vi "Tets.vi"() -> ()   [LabVIEW 2025]
panel:
  in  "Color Box 3":u32(colorbox)
  in  "Color Box 2":u32(colorbox)
  in  "Color Box":u32(colorbox)
  in  "stop":bool
  in  "VISA resource name":refnum<visa-resource-name>
  in  "error in (no error)":errorcluster
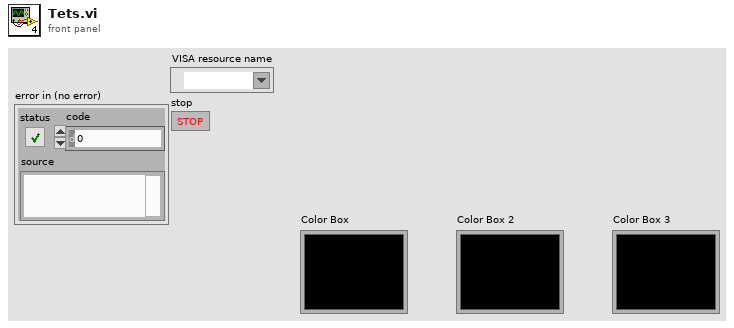
[diagram p1: front panel]
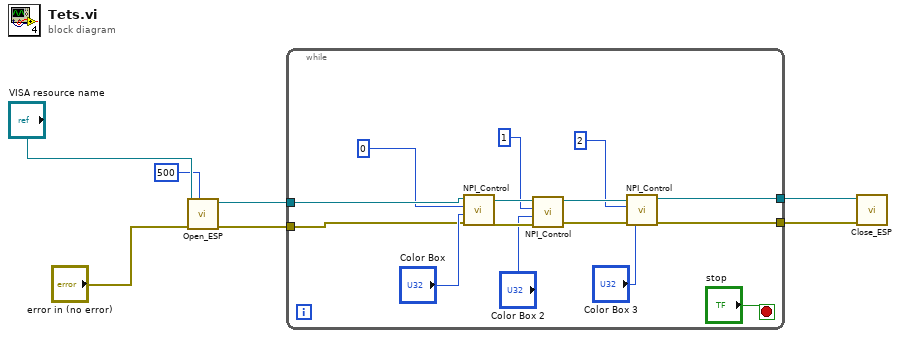
[diagram p0: block diagram]
diagram:
  n1 = call "Open_ESP.vi"("timeout (10sec)"=u32 500, "error in (no error)"="error in (no error)", "VISA resource name"="VISA resource name") -> ("error out"=w3:errorcluster, "VISA resource name out"=w4:refnum<visa-resource-name>)  [unwired: 7 in]
  n2 = while {
    tunnel: w4 -> [w19]
    tunnel: w3 -> [w20]
    tunnel: [w13] -> w2
    tunnel: [w12] -> w1
    stop <- "stop" stop-if-true
    n3 = call "NPI_Control.vi"("error in (no error)"=w20, "Color Box"="Color Box", "No. NeoPixel"=u8 0, "VISA resource name"=w19) -> ("error out"=w16:errorcluster, "VISA resource name out"=w17:refnum<visa-resource-name>)  [unwired: 6 in]
    n4 = call "NPI_Control.vi"("error in (no error)"=w16, "Color Box"="Color Box 2", "No. NeoPixel"=u8 1, "VISA resource name"=w17) -> ("error out"=w11:errorcluster, "VISA resource name out"=w10:refnum<visa-resource-name>)  [unwired: 6 in]
    n5 = call "NPI_Control.vi"("error in (no error)"=w11, "Color Box"="Color Box 3", "No. NeoPixel"=u8 2, "VISA resource name"=w10) -> ("error out"=w12:errorcluster, "VISA resource name out"=w13:refnum<visa-resource-name>)  [unwired: 6 in]
  }
  n6 = call "Close_ESP.vi"("error in (no error)"=w1, "VISA resource name"=w2) -> ()  [unwired: 9 in, 1 out]
